vi "create_pattern.vi"(8 "error in (no error)":errorcluster, 11 "StimulatorDL090503 in":refnum<class "StimulatorDL090503.lvclass">) -> (0 "error out":errorcluster, 3 "StimulatorDL090503 out":refnum<class "StimulatorDL090503.lvclass">)   [LabVIEW 2010, in "StimulatorDL090503.lvclass"]
uses:
  StimulatorDL090503.lvclass
  common/enumerations/functional_global_action_enum.ctl
  StimulatorDL090503.lvclass/StimulatorDL090503.ctl
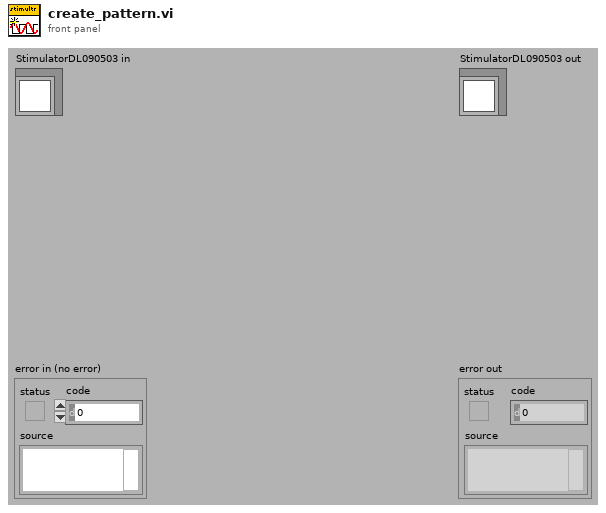
[diagram p1: front panel]
types:
  T1 = typedef "functional_global_action_enum.ctl" = enum16{"get", "set", "reset"}
  T2 = typedef "StimulatorDL090503.lvclass/pattern_type_enum.ctl" = enum16{"sine", "square (+/-)", "square (+)", "square (-)"}
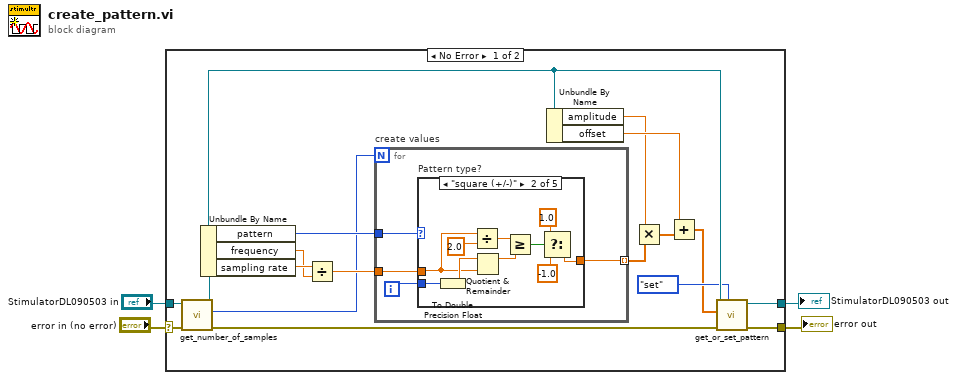
[diagram p0: block diagram]
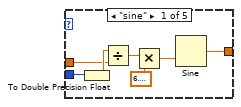
[diagram p2: hidden frame]
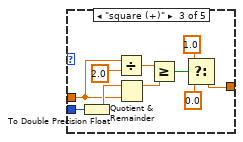
[diagram p3: hidden frame]
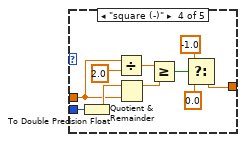
[diagram p4: hidden frame]
diagram:
  n1 = case shown="No Error" "error in (no error)" {
    selector: "error in (no error)" -> [w13 w64]
    tunnel: [w10 w64] -> w3
    tunnel: [w9 w63] -> w4
    tunnel: "StimulatorDL090503 in" -> [w12 w63]
    frame No Error {
      n2 = call "get_number_of_samples.vi"("error in (no error)"=w13, "StimulatorDL090503 in"=w12) -> ("error out"=w11:errorcluster, "number of samples"=w5:i32, "StimulatorDL090503 out"=w8:refnum<class "StimulatorDL090503.lvclass">)  [unwired: 7 in]
      n3 = Unbundle By Name(w8) -> ("pattern"=w18:T2, "frequency"=w19:dbl[unit], "sampling rate"=w21:dbl[unit])
      n4 = Divide(x=w21, y=w19) -> (x/y=w20:dbl)
      n5 = for "create values" {
        N: w5 -> [_]
        tunnel: w18 -> [w25]
        tunnel: [w22] -> w16 mode=indexing
        tunnel: w20 -> [w23]
        i -> [w24]
        n6 = case "Pattern type?" shown="\"square (+/-)\"" w25 {
          tunnel: [w32 w35 w43 w55 _] -> w22
          tunnel: w24 -> [w28 w34 w44 w54 _]
          tunnel: w23 -> [w27 w33 w45 w53 _]
          frame "sine" {
            n7 = To Double Precision Float(number=w28) -> (double precision float=w31:dbl)
            n8 = Divide(x=w31, y=w27) -> (x/y=w30:dbl)
            n9 = Multiply(x=w30, y=6.283185307179586) -> (x*y=w26:dbl)
            n10 = Sine(x=w26) -> (sin(x)=w32:dbl)
          }
          frame "square (+/-)" {
            n11 = To Double Precision Float(number=w34) -> (double precision float=w36:dbl)
            n12 = Divide(x=w33, y=2.0) -> (x/y=w38:dbl)
            n13 = Quotient & Remainder(x=w36, y=w33) -> (x-y*floor(x/y)=w42:dbl)  [unwired: 1 out]
            n14 = Greater Or Equal?(x=w38, y=w42) -> (x >= y?=w39:bool)
            n15 = Select(t=1.0, s=w39, f=-1.0) -> (s? t:f=w35:dbl)
          }
          frame "square (+)" {
            n16 = To Double Precision Float(number=w44) -> (double precision float=w46:dbl)
            n17 = Divide(x=w45, y=2.0) -> (x/y=w48:dbl)
            n18 = Quotient & Remainder(x=w46, y=w45) -> (x-y*floor(x/y)=w52:dbl)  [unwired: 1 out]
            n19 = Greater Or Equal?(x=w48, y=w52) -> (x >= y?=w49:bool)
            n20 = Select(t=1.0, s=w49, f=0.0) -> (s? t:f=w43:dbl)
          }
          frame "square (-)" {
            n21 = To Double Precision Float(number=w54) -> (double precision float=w56:dbl)
            n22 = Divide(x=w53, y=2.0) -> (x/y=w58:dbl)
            n23 = Quotient & Remainder(x=w56, y=w53) -> (x-y*floor(x/y)=w60:dbl)  [unwired: 1 out]
            n24 = Greater Or Equal?(x=w58, y=w60) -> (x >= y?=w59:bool)
            n25 = Select(t=-1.0, s=w59, f=0.0) -> (s? t:f=w55:dbl)
          }
          frame Default {
          }
        }
      }
      n26 = Unbundle By Name(w8) -> ("amplitude"=w14:dbl, "offset"=w17:dbl)
      n27 = Multiply(x=w14, y=w16) -> (x*y=w15:dbl[])
      n28 = Add(x=w17, y=w15) -> (x+y=w6:dbl[])
      n29 = call "get_or_set_pattern.vi"("action"=functional_global_action_enum."set", "error in (no error)"=w11, "pattern in"=w6, "StimulatorDL090503 in"=w8) -> ("error out"=w10:errorcluster, "StimulatorDL090503 out"=w9:refnum<class "StimulatorDL090503.lvclass">)  [unwired: 5 in, 1 out]
    }
    frame Error {
    }
  }
  "error out" <- w3
  "StimulatorDL090503 out" <- w4
